vi "choose firs acquisition state.vi"(8 "error in (no error)":errorcluster, 11 "Channel in":refnum<class "Channel.lvclass">) -> (0 "error out":errorcluster, 2 "verify S4ICS status":bool, 3 "Channel out":refnum<class "Channel.lvclass">)   [LabVIEW 2018, in "Channel.lvclass"]
uses:
  Channel.lvclass
  Channel.lvclass/Channel.ctl
  Header content/Header content.lvclass/Header content.ctl
  Server/Server.lvclass/Server.ctl
  Server/Server.lvclass
  RxTx/CCS_RxTx.lvclass
  Header content/Header content.lvclass
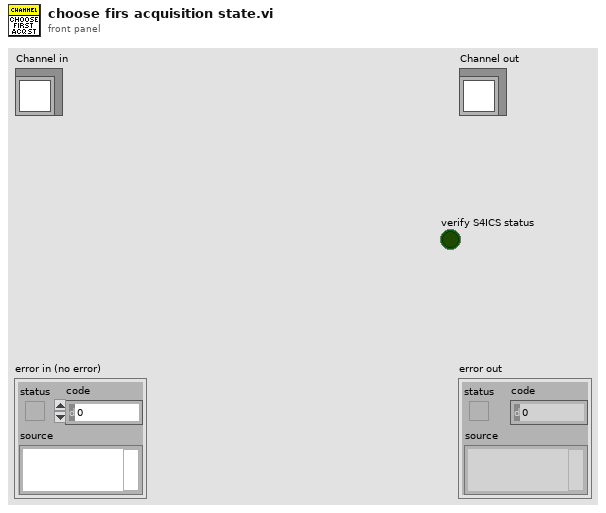
[diagram p1: front panel]
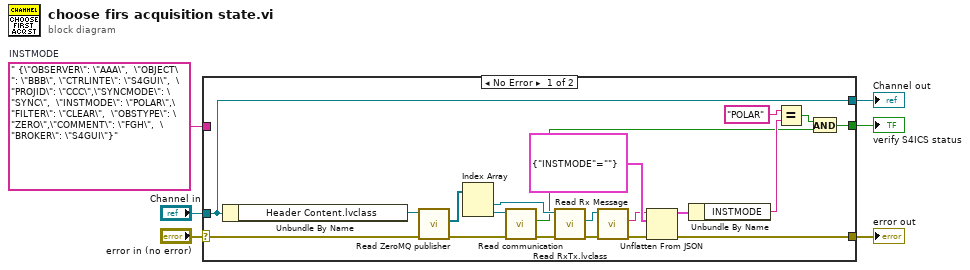
[diagram p0: block diagram]
diagram:
  w2 = " {\"OBSERVER\": \"AAA\",  \"OBJECT\": \"BBB\", \"CTRLINTE\": \"S4GUI\",  \"PROJID\": \"CCC\",\"SYNCMODE\": \"SYNC\",  \"INSTMODE\": \"POLAR\",\"FILTER\": \"CLEAR\",  \"OBSTYPE\": \"ZERO\",\"COMMENT\": \"FGH\",  \"BROKER\": \"S4GUI\"}"  # INSTMODE
  n1 = case shown="No Error" "error in (no error)" {
    selector: "error in (no error)" -> [w21 w28]
    tunnel: [w17 w28] -> w5
    tunnel: [w23 w27] -> w3
    tunnel: "Channel in" -> [w23 w27]
    tunnel: w2 -> [_ _]
    tunnel: [w7 _] -> w1
    frame No Error {
      n2 = Unbundle By Name(w23) -> ("Header Content.lvclass"=w22:refnum<class "Header content.lvclass">)
      n3 = call "Read ZeroMQ publisher.vi"("error in (no error)"=w21, "Header content in"=w22) -> ("error out"=w10:errorcluster, "ZeroMQ publisher"=w26:refnum<class "Server.lvclass">[])  [unwired: 7 in, 1 out]
      n4 = Index Array(array=w26) -> (element #1=w13:refnum<class "Server.lvclass">, element #2=w12:refnum<class "Server.lvclass">)  [unwired: 2 in]
      n5 = call "Read communication.vi"("error in (no error)"=w10, "Server in"=w12) -> ("error out"=w11:errorcluster, "communication"=w8:bool)  [unwired: 7 in, 1 out]
      n6 = call "Read RxTx.lvclass.vi"("error in (no error)"=w11, "Server in"=w13) -> ("error out"=w24:errorcluster, "RxTx.lvclass"=w25:refnum<class "CCS_RxTx.lvclass">)  [unwired: 7 in, 1 out]
      n7 = call "Read Rx Message.vi"("error in (no error)"=w24, "RxTx in"=w25) -> ("error out"=w20:errorcluster, "Rx Message"=w9:string)  [unwired: 7 in, 1 out]
      n8 = Unflatten From JSON(JSON string=w9, type and defaults=cluster{"INSTMODE":string} {"INSTMODE"=""}, error in (no error)=w20) -> (value=w19:cluster{"INSTMODE":string}, error out=w17:errorcluster)  [unwired: 4 in]
      n9 = Unbundle By Name(w19) -> ("INSTMODE"=w16:string)
      n10 = Equal?(x="POLAR", y=w16) -> (x = y?=w14:bool)
      n11 = And(x=w14, y=w8) -> (x .and. y?=w7:bool)
    }
    frame Error {
    }
  }
  "error out" <- w5
  "Channel out" <- w3
  "verify S4ICS status" <- w1
